vi "canDataSort.vi"() -> ()   [LabVIEW 2023] (continued)
\tFF\tFD\r\n      4002  0CF101A7   00000004    8        68\t00\t97\tCC\t00\t19\t39\tE2\r\n      4002  1FFFFFFF   00000004    8        00\t00\tFF\tFF\tFF\tFF\tFF\tFF\r\n      3993  18F106A7   00000004    8        00\tF7\tFF\tFF\tFF\tFF\tFF\tC0\r\n      3992  1FFFFFFF   00000004    8        00\t00\tFF\tFF\tFF\tFF\tFF\tFF\r\n      3983  0CF102A7   00000004    8        30\t75\tE0\t2E\t80\tFF\tFF\tFD\r\n      3983  0CF101A7   00000004    8        68\t00\t97\tCC\t00\t19\t39\tE1\r\n      3982  1FFFFFFF   00000004    8        00\t00\tFF\tFF\tFF\tFF\tFF\tFF\r\n      3972  1FFFFFFF   00000004    8        00\t00\tFF\tFF\tFF\tFF\tFF\tFF\r\n      3963  0CF102A7   00000004    8        30\t75\tE0\t2E\t80\tFF\tFF\tFD\r\n      4022  1FFFFFFF   00000004    8        00\t00\tFF\tFF\tFF\tFF\tFF\tFF\r\n      4012  1FFFFFFF   00000004    8        00\t20\tFF\tFF\tFF\tFF\tFF\tFF\r\n      4003  0CF102A7   00000004    8        30\t75\tE0\t2E\t80\tFF\tFF\tFD\r\n      4002  0CF101A7   00000004    8        68\t00\t97\tCC\t00\t19\t39\tE2\r\n      4002  1FFFFFFF   00000004    8        00\t00\tFF\tFF\tFF\tFF\tFF\tFF\r\n      3993  18F106A7   00000004    8        00\tF7\tFF\tFF\tFF\tFF\tFF\tC0\r\n      3992  1FFFFFFF   00000004    8        00\t00\tFF\tFF\tFF\tFF\tFF\tFF\r\n      3983  0CF102A7   00000004    8        30\t75\tE0\t2E\t80\tFF\tFF\tFD\r\n      3983  0CF101A7   00000004    8        68\t00\t97\tCC\t00\t19\t39\tE1\r\n      3982  1FFFFFFF   00000004    8        00\t00\tFF\tFF\tFF\tFF\tFF\tFF\r\n      3972  1FFFFFFF   00000004    8        00\t00\tFF\tFF\tFF\tFF\tFF\tFF\r\n      4023  0CF101A7   00000004    8        68\t00\t97\tCC\t00\t19\t39\tE3\r\n      4022  1FFFFFFF   00000004    8        00\t00\tFF\tFF\tFF\tFF\tFF\tFF\r\n      4012  1FFFFFFF   00000004    8        00\t20\tFF\tFF\tFF\tFF\tFF\tFF\r\n      4003  0CF102A7   00000004    8        30\t75\tE0\t2E\t80\tFF\tFF\tFD\r\n      4002  0CF101A7   00000004    8        68\t00\t97\tCC\t00\t19\t39\tE2\r\n      4002  1FFFFFFF   00000004    8        00\t00\tFF\tFF\tFF\tFF\tFF\tFF\r\n      3993  18F106A7   00000004    8        00\tF7\tFF\tFF\tFF\tFF\tFF\tC0\r\n      3992  1FFFFFFF   00000004    8        00\t00\tFF\tFF\tFF\tFF\tFF\tFF\r\n      3983  0CF102A7   00000004    8        30\t75\tE0\t2E\t80\tFF\tFF\tFD\r\n      3983  0CF101A7   00000004    8        68\t00\t97\tCC\t00\t19\t39\tE1\r\n      3982  1FFFFFFF   00000004    8        00\t00\tFF\tFF\tFF\tFF\tFF\tFF\r\n      4023  0CF102A7   00000004    8        30\t75\tE0\t2E\t80\tFF\tFF\tFD\r\n      4023  0CF101A7   00000004    8        68\t00\t97\tCC\t00\t19\t39\tE3\r\n      4022  1FFFFFFF   00000004    8        00\t00\tFF\tFF\tFF\tFF\tFF\tFF\r\n      4012  1FFFFFFF   00000004    8        00\t20\tFF\tFF\tFF\tFF\tFF\tFF\r\n      4003  0CF102A7   00000004    8        30\t75\tE0\t2E\t80\tFF\tFF\tFD\r\n      4002  0CF101A7   00000004    8        68\t00\t97\tCC\t00\t19\t39\tE2\r\n      4002  1FFFFFFF   00000004    8        00\t00\tFF\tFF\tFF\tFF\tFF\tFF\r\n      3993  18F106A7   00000004    8        00\tF7\tFF\tFF\tFF\tFF\tFF\tC0\r\n      3992  1FFFFFFF   00000004    8        00\t00\tFF\tFF\tFF\tFF\tFF\tFF\r\n      3983  0CF102A7   00000004    8        30\t75\tE0\t2E\t80\tFF\tFF\tFD\r\n      3983  0CF101A7   00000004    8        68\t00\t97\tCC\t00\t19\t39\tE1\r\n      4032  1FFFFFFF   00000004    8        00\t00\tFF\tFF\tFF\tFF\tFF\tFF\r\n      4023  0CF102A7   00000004    8        30\t75\tE0\t2E\t80\tFF\tFF\tFD\r\n      4023  0CF101A7   00000004    8        68\t00\t97\tCC\t00\t19\t39\tE3\r\n      4022  1FFFFFFF   00000004    8        00\t00\tFF\tFF\tFF\tFF\tFF\tFF\r\n      4012  1FFFFFFF   00000004    8        00\t20\tFF\tFF\tFF\tFF\tFF\tFF\r\n      4003  0CF102A7   00000004    8        30\t75\tE0\t2E\t80\tFF\tFF\tFD\r\n      4002  0CF101A7   00000004    8        68\t00\t97\tCC\t00\t19\t39\tE2\r\n      4002  1FFFFFFF   00000004    8        00\t00\tFF\tFF\tFF\tFF\tFF\tFF\r\n      3993  18F106A7   00000004    8        00\tF7\tFF\tFF\tFF\tFF\tFF\tC0\r\n      3992  1FFFFFFF   00000004    8        00\t00\tFF\tFF\tFF\tFF\tFF\tFF\r\n      3983  0CF102A7   00000004    8        30\t75\tE0\t2E\t80\tFF\tFF\tFD\r\n      4041  18F11FF0   00000004    8        FF\t3F\t90\t68\t88\t1B\t10\t0C\r\n      4032  1FFFFFFF   00000004    8        00\t00\tFF\tFF\tFF\tFF\tFF\tFF\r\n      4023  0CF102A7   00000004    8        30\t75\tE0\t2E\t80\tFF\tFF\tFD\r\n      4023  0CF101A7   00000004    8        68\t00\t97\tCC\t00\t19\t39\tE3\r\n      4022  1FFFFFFF   00000004    8        00\t00\tFF\tFF\tFF\tFF\tFF\tFF\r\n      4012  1FFFFFFF   00000004    8        00\t20\tFF\tFF\tFF\tFF\tFF\tFF\r\n      4003  0CF102A7   00000004    8        30\t75\tE0\t2E\t80\tFF\tFF\tFD\r\n      4002  0CF101A7   00000004    8        68\t00\t97\tCC\t00\t19\t39\tE2\r\n      4002  1FFFFFFF   00000004    8        00\t00\tFF\tFF\tFF\tFF\tFF\tFF\r\n      3993  18F106A7   00000004    8        00\tF7\tFF\tFF\tFF\tFF\tFF\tC0\r\n      3992  1FFFFFFF   00000004    8        00\t00\tFF\tFF\tFF\tFF\tFF\tFF\r\n      4042  18F120F0   00000004    8        2B\t75\t60\tB1\tB0\t01\tFF\tFF\r\n      4041  18F11FF0   00000004    8        FF\t3F\t90\t68\t88\t1B\t10\t0C\r\n      4032  1FFFFFFF   00000004    8        00\t00\tFF\tFF\tFF\tFF\tFF\tFF\r\n      4023  0CF102A7   00000004    8        30\t75\tE0\t2E\t80\tFF\tFF\tFD\r\n      4023  0CF101A7   00000004    8        68\t00\t97\tCC\t00\t19\t39\tE3\r\n      4022  1FFFFFFF   00000004    8        00\t00\tFF\tFF\tFF\tFF\tFF\tFF\r\n      4012  1FFFFFFF   00000004    8        00\t20\tFF\tFF\tFF\tFF\tFF\tFF\r\n      4003  0CF102A7   00000004    8        30\t75\tE0\t2E\t80\tFF\tFF\tFD\r\n      4002  0CF101A7   00000004    8        68\t00\t97\tCC\t00\t19\t39\tE2\r\n      4002  1FFFFFFF   00000004    8        00\t00\tFF\tFF\tFF\tFF\tFF\tFF\r\n      3993  18F106A7   00000004    8        00\tF7\tFF\tFF\tFF\tFF\tFF\tC0\r\n      4043  0CF101A7   00000004    8        68\t00\t97\tCC\t00\t19\t39\tE4\r\n      4042  18F120F0   00000004    8        2B\t75\t60\tB1\tB0\t01\tFF\tFF\r\n      4041  18F11FF0   00000004    8        FF\t3F\t90\t68\t88\t1B\t10\t0C\r\n      4032  1FFFFFFF   00000004    8        00\t00\tFF\tFF\tFF\tFF\tFF\tFF\r\n      4023  0CF102A7   00000004    8        30\t75\tE0\t2E\t80\tFF\tFF\tFD\r\n      4023  0CF101A7   00000004    8        68\t00\t97\tCC\t00\t19\t39\tE3\r\n      4022  1FFFFFFF   00000004    8        00\t00\tFF\tFF\tFF\tFF\tFF\tFF\r\n      4012  1FFFFFFF   00000004    8        00\t20\tFF\tFF\tFF\tFF\tFF\tFF\r\n      4003  0CF102A7   00000004    8        30\t75\tE0\t2E\t80\tFF\tFF\tFD\r\n      4002  0CF101A7   00000004    8        68\t00\t97\tCC\t00\t19\t39\tE2\r\n      4002  1FFFFFFF   00000004    8        00\t00\tFF\tFF\tFF\tFF\tFF\tFF\r\n      4043  0C3C4D4A   00000004    8        BE\tFF\tFF\t7F\t18\tFF\tFF\t60\r\n      4043  0CF101A7   00000004    8        68\t00\t97\tCC\t00\t19\t39\tE4\r\n      4042  18F120F0   00000004    8        2B\t75\t60\tB1\tB0\t01\tFF\tFF\r\n      4041  18F11FF0   00000004    8        FF\t3F\t90\t68\t88\t1B\t10\t0C\r\n      4032  1FFFFFFF   00000004    8        00\t00\tFF\tFF\tFF\tFF\tFF\tFF\r\n      4023  0CF102A7   00000004    8        30\t75\tE0\t2E\t80\tFF\tFF\tFD\r\n      4023  0CF101A7   00000004    8        68\t00\t97\tCC\t00\t19\t39\tE3\r\n      4022  1FFFFFFF   00000004    8        00\t00\tFF\tFF\tFF\tFF\tFF\tFF\r\n      4012  1FFFFFFF   00000004    8        00\t20\tFF\tFF\tFF\tFF\tFF\tFF\r\n      4003  0CF102A7   00000004    8        30\t75\tE0\t2E\t80\tFF\tFF\tFD\r\n      4002  0CF101A7   00000004    8        68\t00\t97\tCC\t00\t19\t39\tE2\r\n      4044  0CF102A7   00000004    8        30\t75\tE0\t2E\t80\tFF\tFF\tFD\r\n      4043  0C3C4D4A   00000004    8        BE\tFF\tFF\t7F\t18\tFF\tFF\t60\r\n      4043  0CF101A7   00000004    8        68\t00\t97\tCC\t00\t19\t39\tE4\r\n      4042  18F120F0   00000004    8        2B\t75\t60\tB1\tB0\t01\tFF\tFF\r\n      4041  18F11FF0   00000004    8        FF\t3F\t90\t68\t88\t1B\t10\t0C\r\n      4032  1FFFFFFF   00000004    8        00\t00\tFF\tFF\tFF\tFF\tFF\tFF\r\n      4023  0CF102A7   00000004    8        30\t75\tE0\t2E\t80\tFF\tFF\tFD\r\n      4023  0CF101A7   00000004    8        68\t00\t97\tCC\t00\t19\t39\tE3\r\n      4022  1FFFFFFF   00000004    8        00\t00\tFF\tFF\tFF\tFF\tFF\tFF\r\n      4012  1FFFFFFF   00000004    8        00\t20\tFF\tFF\tFF\tFF\tFF\tFF\r\n      4003  0CF102A7   00000004    8        30\t75\tE0\t2E\t80\tFF\tFF\tFD\r\n      4044  0CF103A7   00000004    8        17\t1F\t08\t60\tB1\t1F\t08\t60\r\n      4044  0CF102A7   00000004    8        30\t75\tE0\t2E\t80\tFF\tFF\tFD\r\n      4043  0C3C4D4A   00000004    8        BE\tFF\tFF\t7F\t18\tFF\tFF\t60\r\n      4043  0CF101A7   00000004    8        68\t00\t97\tCC\t00\t19\t39\tE4\r\n      4042  18F120F0   00000004    8        2B\t75\t60\tB1\tB0\t01\tFF\tFF\r\n      4041  18F11FF0   00000004    8        FF\t3F\t90\t68\t88\t1B\t10\t0C\r\n      4032  1FFFFFFF   00000004    8        00\t00\tFF\tFF\tFF\tFF\tFF\tFF\r\n      4023  0CF102A7   00000004    8        30\t75\tE0\t2E\t80\tFF\tFF\tFD\r\n      4023  0CF101A7   00000004    8        68\t00\t97\tCC\t00\t19\t39\tE3\r\n      4022  1FFFFFFF   00000004    8        00\t00\tFF\tFF\tFF\tFF\tFF\tFF\r\n      4012  1FFFFFFF   00000004    8        00\t20\tFF\tFF\tFF\tFF\tFF\tFF\r\n      4045  0CF104A7   00000004    8        F0\t60\t22\tFC\tFF\tFF\tFF\t60\r\n      4044  0CF103A7   00000004    8        17\t1F\t08\t60\tB1\t1F\t08\t60\r\n      4044  0CF102A7   00000004    8        30\t75\tE0\t2E\t80\tFF\tFF\tFD\r\n      4043  0C3C4D4A   00000004    8        BE\tFF\tFF\t7F\t18\tFF\tFF\t60\r\n      4043  0CF101A7   00000004    8        68\t00\t97\tCC\t00\t19\t39\tE4\r\n      4042  18F120F0   00000004    8        2B\t75\t60\tB1\tB0\t01\tFF\tFF\r\n      4041  18F11FF0   00000004    8        FF\t3F\t90\t68\t88\t1B\t10\t0C\r\n      4032  1FFFFFFF   00000004    8        00\t00\tFF\tFF\tFF\tFF\tFF\tFF\r\n      4023  0CF102A7   00000004    8        30\t75\tE0\t2E\t80\tFF\tFF\tFD\r\n      4023  0CF101A7   00000004    8        68\t00\t97\tCC\t00\t19\t39\tE3\r\n      4022  1FFFFFFF   00000004    8        00\t00\tFF\tFF\tFF\tFF\tFF\tFF\r\n      4045  18F106A7   00000004    8        00\tF7\tFF\tFF\tFF\tFF\tFF\tC1\r\n      4045  0CF104A7   00000004    8        F0\t60\t22\tFC\tFF\tFF\tFF\t60\r\n      4044  0CF103A7   00000004    8        17\t1F\t08\t60\tB1\t1F\t08\t60\r\n      4044  0CF102A7   00000004    8        30\t75\tE0\t2E\t80\tFF\tFF\tFD\r\n      4043  0C3C4D4A   00000004    8        BE\tFF\tFF\t7F\t18\tFF\tFF\t60\r\n      4043  0CF101A7   00000004    8        68\t00\t97\tCC\t00\t19\t39\tE4\r\n      4042  18F120F0   00000004    8        2B\t75\t60\tB1\tB0\t01\tFF\tFF\r\n      4041  18F11FF0   00000004    8        FF\t3F\t90\t68\t88\t1B\t10\t0C\r\n      4032  1FFFFFFF   00000004    8        00\t00\tFF\tFF\tFF\tFF\tFF\tFF\r\n      4023  0CF102A7   00000004    8        30\t75\tE0\t2E\t80\tFF\tFF\tFD\r\n      4023  0CF101A7   00000004    8        68\t00\t97\tCC\t00\t19\t39\tE3\r\n      4046  18F121F0   00000004    8        09\t34\t00\t00\tFF\tFF\tB0\t01\r\n      4045  18F106A7   00000004    8        00\tF7\tFF\tFF\tFF\tFF\tFF\tC1\r\n      4045  0CF104A7   00000004    8        F0\t60\t22\tFC\tFF\tFF\tFF\t60\r\n      4044  0CF103A7   00000004    8        17\t1F\t08\t60\tB1\t1F\t08\t60\r\n      4044  0CF102A7   00000004    8        30\t75\tE0\t2E\t80\tFF\tFF\tFD\r\n      4043  0C3C4D4A   00000004    8        BE\tFF\tFF\t7F\t18\tFF\tFF\t60\r\n      4043  0CF101A7   00000004    8        68\t00\t97\tCC\t00\t19\t39\tE4\r\n      4042  18F120F0   00000004    8        2B\t75\t60\tB1\tB0\t01\tFF\tFF\r\n      4041  18F11FF0   00000004    8        FF\t3F\t90\t68\t88\t1B\t10\t0C\r\n      4032  1FFFFFFF   00000004    8        00\t00\tFF\tFF\tFF\tFF\tFF\tFF\r\n      4023  0CF102A7   00000004    8        30\t75\tE0\t2E\t80\tFF\tFF\tFD\r\n      4047  1FFFFFFF   00000004    8        00\t00\tFF\tFF\tFF\tFF\tFF\tFF\r\n      4046  18F121F0   00000004    8        09\t34\t00\t00\tFF\tFF\tB0\t01\r\n      4045  18F106A7   00000004    8        00\tF7\tFF\tFF\tFF\tFF\tFF\tC1\r\n      4045  0CF104A7   00000004    8        F0\t60\t22\tFC\tFF\tFF\tFF\t60\r\n      4044  0CF103A7   00000004    8        17\t1F\t08\t60\tB1\t1F\t08\t60\r\n      4044  0CF102A7   00000004    8        30\t75\tE0\t2E\t80\tFF\tFF\tFD\r\n      4043  0C3C4D4A   00000004    8        BE\tFF\tFF\t7F\t18\tFF\tFF\t60\r\n      4043  0CF101A7   00000004    8        68\t00\t97\tCC\t00\t19\t39\tE4\r\n      4042  18F120F0   00000004    8        2B\t75\t60\tB1\tB0\t01\tFF\tFF\r\n      4041  18F11FF0   00000004    8        FF\t3F\t90\t68\t88\t1B\t10\t0C\r\n      4032  1FFFFFFF   00000004    8        00\t00\tFF\tFF\tFF\tFF\tFF\tFF\r\n      4052  1FFFFFFF   00000004    8        00\t20\tFF\tFF\tFF\tFF\tFF\tFF\r\n      4047  1FFFFFFF   00000004    8        00\t00\tFF\tFF\tFF\tFF\tFF\tFF\r\n      4046  18F121F0   00000004    8        09\t34\t00\t00\tFF\tFF\tB0\t01\r\n      4045  18F106A7   00000004    8        00\tF7\tFF\tFF\tFF\tFF\tFF\tC1\r\n      4045  0CF104A7   00000004    8        F0\t60\t22\tFC\tFF\tFF\tFF\t60\r\n      4044  0CF103A7   00000004    8        17\t1F\t08\t60\tB1\t1F\t08\t60\r\n      4044  0CF102A7   00000004    8        30\t75\tE0\t2E\t80\tFF\tFF\tFD\r\n      4043  0C3C4D4A   00000004    8        BE\tFF\tFF\t7F\t18\tFF\tFF\t60\r\n      4043  0CF101A7   00000004    8        68\t00\t97\tCC\t00\t19\t39\tE4\r\n      4042  18F120F0   00000004    8        2B\t75\t60\tB1\tB0\t01\tFF\tFF\r\n      4041  18F11FF0   00000004    8        FF\t3F\t90\t68\t88\t1B\t10\t0C\r\n      4062  1FFFFFFF   00000004    8        00\t00\tFF\tFF\tFF\tFF\tFF\tFF\r\n      4052  1FFFFFFF   00000004    8        00\t20\tFF\tFF\tFF\tFF\tFF\tFF\r\n      4047  1FFFFFFF   00000004    8        00\t00\tFF\tFF\tFF\tFF\tFF\tFF\r\n      4046  18F121F0   00000004    8        09\t34\t00\t00\tFF\tFF\tB0\t01\r\n      4045  18F106A7   00000004    8        00\tF7\tFF\tFF\tFF\tFF\tFF\tC1\r\n      4045  0CF104A7   00000004    8        F0\t60\t22\tFC\tFF\tFF\tFF\t60\r\n      4044  0CF103A7   00000004    8        17\t1F\t08\t60\tB1\t1F\t08\t60\r\n      4044  0CF102A7   00000004    8        30\t75\tE0\t2E\t80\tFF\tFF\tFD\r\n      4043  0C3C4D4A   00000004    8        BE\tFF\tFF\t7F\t18\tFF\tFF\t60\r\n      4043  0CF101A7   00000004    8        68\t00\t97\tCC\t00\t19\t39\tE4\r\n      4042  18F120F0   00000004    8        2B\t75\t60\tB1\tB0\t01\tFF\tFF\r\n      4063  0CF101A7   00000004    8        68\t00\t97\tCC\t00\t19\t39\tE5\r\n      4062  1FFFFFFF   00000004    8        00\t00\tFF\tFF\tFF\tFF\tFF\tFF\r\n      4052  1FFFFFFF   00000004    8        00\t20\tFF\tFF\tFF\tFF\tFF\tFF\r\n      4047  1FFFFFFF   00000004    8        00\t00\tFF\tFF\tFF\tFF\tFF\tFF\r\n      4046  18F121F0   00000004    8        09\t34\t00\t00\tFF\tFF\tB0\t01\r\n      4045  18F106A7   00000004    8        00\tF7\tFF\tFF\tFF\tFF\tFF\tC1\r\n      4045  0CF104A7   00000004    8        F0\t60\t22\tFC\tFF\tFF\tFF\t60\r\n      4044  0CF103A7   00000004    8        17\t1F\t08\t60\tB1\t1F\t08\t60\r\n      4044  0CF102A7   00000004    8        30\t75\tE0\t2E\t80\tFF\tFF\tFD\r\n      4043  0C3C4D4A   00000004    8        BE\tFF\tFF\t7F\t18\tFF\tFF\t60\r\n      4043  0CF101A7   00000004    8        68\t00\t97\tCC\t00\t19\t39\tE4\r\n      4063  0CF102A7   00000004    8        30\t75\tE0\t2E\t80\tFF\tFF\tFD\r\n      4063  0CF101A7   00000004    8        68\t00\t97\tCC\t00\t19\t39\tE5\r\n      4062  1FFFFFFF   00000004    8        00\t00\tFF\tFF\tFF\tFF\tFF\tFF\r\n      4052  1FFFFFFF   00000004    8        00\t20\tFF\tFF\tFF\tFF\tFF\tFF\r\n      4047  1FFFFFFF   00000004    8        00\t00\tFF\tFF\tFF\tFF\tFF\tFF\r\n      4046  18F121F0   00000004    8        09\t34\t00\t00\tFF\tFF\tB0\t01\r\n      4045  18F106A7   00000004    8        00\tF7\tFF\tFF\tFF\tFF\tFF\tC1\r\n      4045  0CF104A7   00000004    8        F0\t60\t22\tFC\tFF\tFF\tFF\t60\r\n      4044  0CF103A7   00000004    8        17\t1F\t08\t60\tB1\t1F\t08\t60\r\n      4044  0CF102A7   00000004    8        30\t75\tE0\t2E\t80\tFF\tFF\tFD\r\n      4043  0C3C4D4A   00000004    8        BE\tFF\tFF\t7F\t18\tFF\tFF\t60\r\n      4072  1FFFFFFF   00000004    8        00\t20\tFF\tFF\tFF\tFF\tFF\tFF\r\n      4063  0CF102A7   00000004    8        30\t75\tE0\t2E\t80\tFF\tFF\tFD\r\n      4063  0CF101A7   00000004    8        68\t00\t97\tCC\t00\t19\t39\tE5\r\n      4062  1FFFFFFF   00000004    8        00\t00\tFF\tFF\tFF\tFF\tFF\tFF\r\n      4052  1FFFFFFF   00000004    8        00\t20\tFF\tFF\tFF\tFF\tFF\tFF\r\n      4047  1FFFFFFF   00000004    8        00\t00\tFF\tFF\tFF\tFF\tFF\tFF\r\n      4046  18F121F0   00000004    8        09\t34\t00\t00\tFF\tFF\tB0\t01\r\n      4045  18F106A7   00000004    8        00\tF7\tFF\tFF\tFF\tFF\tFF\tC1\r\n      4045  0CF104A7   00000004    8        F0\t60\t22\tFC\tFF\tFF\tFF\t60\r\n      4044  0CF103A7   00000004    8        17\t1F\t08\t60\tB1\t1F\t08\t60\r\n      4044  0CF102A7   00000004    8        30\t75\tE0\t2E\t80\tFF\tFF\tFD\r\n      4082  1FFFFFFF   00000004    8        00\t20\tFF\tFF\tFF\tFF\tFF\tFF\r\n      4072  1FFFFFFF   00000004    8        00\t20\tFF\tFF\tFF\tFF\tFF\tFF\r\n      4063  0CF102A7   00000004    8        30\t75\tE0\t2E\t80\tFF\tFF\tFD\r\n      4063  0CF101A7   00000004    8        68\t00\t97\tCC\t00\t19\t39\tE5\r\n      4062  1FFFFFFF   00000004    8        00\t00\tFF\tFF\tFF\tFF\tFF\tFF\r\n      4052  1FFFFFFF   00000004    8        00\t20\tFF\tFF\tFF\tFF\tFF\tFF\r\n      4047  1FFFFFFF   00000004    8        00\t00\tFF\tFF\tFF\tFF\tFF\tFF\r\n      4046  18F121F0   00000004    8        09\t34\t00\t00\tFF\tFF\tB0\t01\r\n      4045  18F106A7   00000004    8        00\tF7\tFF\tFF\tFF\tFF\tFF\tC1\r\n      4045  0CF104A7   00000004    8        F0\t60\t22\tFC\tFF\tFF\tFF\t60\r\n      4044  0CF103A7   00000004    8        17\t1F\t08\t60\tB1\t1F\t08\t60\r\n      4083  0CF101A7   00000004    8        68\t00\t97\tCC\t00\t19\t39\tE6\r\n      4082  1FFFFFFF   00000004    8        00\t20\tFF\tFF\tFF\tFF\tFF\tFF\r\n      4072  1FFFFFFF   00000004    8        00\t20\tFF\tFF\tFF\tFF\tFF\tFF\r\n      4063  0CF102A7   00000004    8        30\t75\tE0\t2E\t80\tFF\tFF\tFD\r\n      4063  0CF101A7   00000004    8        68\t00\t97\tCC\t00\t19\t39\tE5\r\n      4062  1FFFFFFF   00000004    8        00\t00\tFF\tFF\tFF\tFF\tFF\tFF\r\n      4052  1FFFFFFF   00000004    8        00\t20\tFF\tFF\tFF\tFF\tFF\tFF\r\n      4047  1FFFFFFF   00000004    8        00\t00\tFF\tFF\tFF\tFF\tFF\tFF\r\n      4046  18F121F0   00000004    8        09\t34\t00\t00\tFF\tFF\tB0\t01\r\n      4045  18F106A7   00000004    8        00\tF7\tFF\tFF\tFF\tFF\tFF\tC1\r\n      4045  0CF104A7   00000004    8        F0\t60\t22\tFC\tFF\tFF\tFF\t60\r\n      4083  0CF102A7   00000004    8        30\t75\tE0\t2E\t80\tFF\tFF\tFD\r\n      4083  0CF101A7   00000004    8        68\t00\t97\tCC\t00\t19\t39\tE6\r\n      4082  1FFFFFFF   00000004    8        00\t20\tFF\tFF\tFF\tFF\tFF\tFF\r\n      4072  1FFFFFFF   00000004    8        00\t20\tFF\tFF\tFF\tFF\tFF\tFF\r\n      4063  0CF102A7   00000004    8        30\t75\tE0\t2E\t80\tFF\tFF\tFD\r\n      4063  0CF101A7   00000004    8        68\t00\t97\tCC\t00\t19\t39\tE5\r\n      4062  1FFFFFFF   00000004    8        00\t00\tFF\tFF\tFF\tFF\tFF\tFF\r\n      4052  1FFFFFFF   00000004    8        00\t20\tFF\tFF\tFF\tFF\tFF\tFF\r\n      4047  1FFFFFFF   00000004    8        00\t00\tFF\tFF\tFF\tFF\tFF\tFF\r\n      4046  18F121F0   00000004    8        09\t34\t00\t00\tFF\tFF\tB0\t01\r\n      4045  18F106A7   00000004    8        00\tF7\tFF\tFF\tFF\tFF\tFF\tC1\r\n      4092  1FFFFFFF   00000004    8        00\t00\tFF\tFF\tFF\tFF\tFF\tFF\r\n      4083  0CF102A7   00000004    8        30\t75\tE0\t2E\t80\tFF\tFF\tFD\r\n      4083  0CF101A7   00000004    8        68\t00\t97\tCC\t00\t19\t39\tE6\r\n      4082  1FFFFFFF   00000004    8        00\t20\tFF\tFF\tFF\tFF\tFF\tFF\r\n      4072  1FFFFFFF   00000004    8        00\t20\tFF\tFF\tFF\tFF\tFF\tFF\r\n      4063  0CF102A7   00000004    8        30\t75\tE0\t2E\t80\tFF\tFF\tFD\r\n      4063  0CF101A7   00000004    8        68\t00\t97\tCC\t00\t19\t39\tE5\r\n      4062  1FFFFFFF   00000004    8        00\t00\tFF\tFF\tFF\tFF\tFF\tFF\r\n      4052  1FFFFFFF   00000004    8        00\t20\tFF\tFF\tFF\tFF\tFF\tFF\r\n      4047  1FFFFFFF   00000004    8        00\t00\tFF\tFF\tFF\tFF\tFF\tFF\r\n      4046  18F121F0   00000004    8        09\t34\t00\t00\tFF\tFF\tB0\t01\r\n      4093  18F106A7   00000004    8        00\tF7\tFF\tFF\tFF\tFF\tFF\tC2\r\n      4092  1FFFFFFF   00000004    8        00\t00\tFF\tFF\tFF\tFF\tFF\tFF\r\n      4083  0CF102A7   00000004    8        30\t75\tE0\t2E\t80\tFF\tFF\tFD\r\n      4083  0CF101A7   00000004    8        68\t00\t97\tCC\t00\t19\t39\tE6\r\n      4082  1FFFFFFF   00000004    8        00\t20\tFF\tFF\tFF\tFF\tFF\tFF\r\n      4072  1FFFFFFF   00000004    8        00\t20\tFF\tFF\tFF\tFF\tFF\tFF\r\n      4063  0CF102A7   00000004    8        30\t75\tE0\t2E\t80\tFF\tFF\tFD\r\n      4063  0CF101A7   00000004    8        68\t00\t97\tCC\t00\t19\t39\tE5\r\n      4062  1FFFFFFF   00000004    8        00\t00\tFF\tFF\tFF\tFF\tFF\tFF\r\n      4052  1FFFFFFF   00000004    8        00\t20\tFF\tFF\tFF\tFF\tFF\tFF\r\n      4047  1FFFFFFF   00000004    8        00\t00\tFF\tFF\tFF\tFF\tFF\tFF\r\n      4102  1FFFFFFF   00000004    8        00\t20\tFF\tFF\tFF\tFF\tFF\tFF\r\n      4093  18F106A7   00000004    8        00\tF7\tFF\tFF\tFF\tFF\tFF\tC2\r\n      4092  1FFFFFFF   00000004    8        00\t00\tFF\tFF\tFF\tFF\tFF\tFF\r\n      4083  0CF102A7   00000004    8        30\t75\tE0\t2E\t80\tFF\tFF\tFD\r\n      4083  0CF101A7   00000004    8        68\t00\t97\tCC\t00\t19\t39\tE6\r\n      4082  1FFFFFFF   00000004    8        00\t20\tFF\tFF\tFF\tFF\tFF\tFF\r\n      4072  1FFFFFFF   00000004    8        00\t20\tFF\tFF\tFF\tFF\tFF\tFF\r\n      4063  0CF102A7   00000004    8        30\t75\tE0\t2E\t80\tFF\tFF\tFD\r\n      4063  0CF101A7   00000004    8        68\t00\t97\tCC\t00\t19\t39\tE5\r\n      4062  1FFFFFFF   00000004    8        00\t00\tFF\tFF\tFF\tFF\tFF\tFF\r\n      4052  1FFFFFFF   00000004    8        00\t20\tFF\tFF\tFF\tFF\tFF\tFF\r\n      4103  0CF101A7   00000004    8        68\t00\t97\tCC\t00\t19\t39\tE7\r\n      4102  1FFFFFFF   00000004    8        00\t20\tFF\tFF\tFF\tFF\tFF\tFF\r\n      4093  18F106A7   00000004    8        00\tF7\tFF\tFF\tFF\tFF\tFF\tC2\r\n      4092  1FFFFFFF   00000004    8        00\t00\tFF\tFF\tFF\tFF\tFF\tFF\r\n      4083  0CF102A7   00000004    8        30\t75\tE0\t2E\t80\tFF\tFF\tFD\r\n      4083  0CF101A7   00000004    8        68\t00\t97\tCC\t00\t19\t39\tE6\r\n      4082  1FFFFFFF   00000004    8        00\t20\tFF\tFF\tFF\tFF\tFF\tFF\r\n      4072  1FFFFFFF   00000004    8        00\t20\tFF\tFF\tFF\tFF\tFF\tFF\r\n      4063  0CF102A7   00000004    8        30\t75\tE0\t2E\t80\tFF\tFF\tFD\r\n      4063  0CF101A7   00000004    8        68\t00\t97\tCC\t00\t19\t39\tE5\r\n      4062  1FFFFFFF   00000004    8        00\t00\tFF\tFF\tFF\tFF\tFF\tFF\r\n      4103  0CF102A7   00000004    8        30\t75\tE0\t2E\t80\tFF\tFF\tFD\r\n      4103  0CF101A7   00000004    8        68\t00\t97\tCC\t00\t19\t39\tE7\r\n      4102  1FFFFFFF   00000004    8        00\t20\tFF\tFF\tFF\tFF\tFF\tFF\r\n      4093  18F106A7   00000004    8        00\tF7\tFF\tFF\tFF\tFF\tFF\tC2\r\n      4092  1FFFFFFF   00000004    8        00\t00\tFF\tFF\tFF\tFF\tFF\tFF\r\n      4083  0CF102A7   00000004    8        30\t75\tE0\t2E\t80\tFF\tFF\tFD\r\n      4083  0CF101A7   00000004    8        68\t00\t97\tCC\t00\t19\t39\tE6\r\n      4082  1FFFFFFF   00000004    8        00\t20\tFF\tFF\tFF\tFF\tFF\tFF\r\n      4072  1FFFFFFF   00000004    8        00\t20\tFF\tFF\tFF\tFF\tFF\tFF\r\n      4063  0CF102A7   00000004    8        30\t75\tE0\t2E\t80\tFF\tFF\tFD\r\n      4063  0CF101A7   00000004    8        68\t00\t97\tCC\t00\t19\t39\tE5\r\n      4112  1FFFFFFF   00000004    8        00\t00\tFF\tFF\tFF\tFF\tFF\tFF\r\n      4103  0CF102A7   00000004    8        30\t75\tE0\t2E\t80\tFF\tFF\tFD\r\n      4103  0CF101A7   00000004    8        68\t00\t97\tCC\t00\t19\t39\tE7\r\n      4102  1FFFFFFF   00000004    8        00\t20\tFF\tFF\tFF\tFF\tFF\tFF\r\n      4093  18F106A7   00000004    8        00\tF7\tFF\tFF\tFF\tFF\tFF\tC2\r\n      4092  1FFFFFFF   00000004    8        00\t00\tFF\tFF\tFF\tFF\tFF\tFF\r\n      4083  0CF102A7   00000004    8        30\t75\tE0\t2E\t80\tFF\tFF\tFD\r\n      4083  0CF101A7   00000004    8        68\t00\t97\tCC\t00\t19\t39\tE6\r\n      4082  1FFFFFFF   00000004    8        00\t20\tFF\tFF\tFF\tFF\tFF\tFF\r\n      4072  1FFFFFFF   00000004    8        00\t20\tFF\tFF\tFF\tFF\tFF\tFF\r\n      4063  0CF102A7   00000004    8        30\t75\tE0\t2E\t80\tFF\tFF\tFD\r\n      4122  1FFFFFFF   00000004    8        00\t20\tFF\tFF\tFF\tFF\tFF\tFF\r\n      4112  1FFFFFFF   00000004    8        00\t00\tFF\tFF\tFF\tFF\tFF\tFF\r\n      4103  0CF102A7   00000004    8        30\t75\tE0\t2E\t80\tFF\tFF\tFD\r\n      4103  0CF101A7   00000004    8        68\t00\t97\tCC\t00\t19\t39\tE7\r\n      4102  1FFFFFFF   00000004    8        00\t20\tFF\tFF\tFF\tFF\tFF\tFF\r\n      4093  18F106A7   00000004    8        00\tF7\tFF\tFF\tFF\tFF\tFF\tC2\r\n      4092  1FFFFFFF   00000004    8        00\t00\tFF\tFF\tFF\tFF\tFF\tFF\r\n      4083  0CF102A7   00000004    8        30\t75\tE0\t2E\t80\tFF\tFF\tFD\r\n      4083  0CF101A7   00000004    8        68\t00\t97\tCC\t00\t19\t39\tE6\r\n      4082  1FFFFFFF   00000004    8        00\t20\tFF\tFF\tFF\tFF\tFF\tFF\r\n      4072  1FFFFFFF   00000004    8        00\t20\tFF\tFF\tFF\tFF\tFF\tFF\r\n      4123  0CF101A7   00000004    8        68\t00\t97\tCC\t00\t19\t39\tE8\r\n      4122  1FFFFFFF   00000004    8        00\t20\tFF\tFF\tFF\tFF\tFF\tFF\r\n      4112  1FFFFFFF   00000004    8        00\t00\tFF\tFF\tFF\tFF\tFF\tFF\r\n      4103  0CF102A7   00000004    8        30\t75\tE0\t2E\t80\tFF\tFF\tFD\r\n      4103  0CF101A7   00000004    8        68\t00\t97\tCC\t00\t19\t39\tE7\r\n      4102  1FFFFFFF   00000004    8        00\t20\tFF\tFF\tFF\tFF\tFF\tFF\r\n      4093  18F106A7   00000004    8        00\tF7\tFF\tFF\tFF\tFF\tFF\tC2\r\n      4092  1FFFFFFF   00000004    8        00\t00\tFF\tFF\tFF\tFF\tFF\tFF\r\n      4083  0CF102A7   00000004    8        30\t75\tE0\t2E\t80\tFF\tFF\tFD\r\n      4083  0CF101A7   00000004    8        68\t00\t97\tCC\t00\t19\t39\tE6\r\n      4082  1FFFFFFF   00000004    8        00\t20\tFF\tFF\tFF\tFF\tFF\tFF\r\n      4123  0CF102A7   00000004    8        30\t75\tE0\t2E\t80\tFF\tFF\tFD\r\n      4123  0CF101A7   00000004    8        68\t00\t97\tCC\t00\t19\t39\tE8\r\n      4122  1FFFFFFF   00000004    8        00\t20\tFF\tFF\tFF\tFF\tFF\tFF\r\n      4112  1FFFFFFF   00000004    8        00\t00\tFF\tFF\tFF\tFF\tFF\tFF\r\n      4103  0CF102A7   00000004    8        30\t75\tE0\t2E\t80\tFF\tFF\tFD\r\n      4103  0CF101A7   00000004    8        68\t00\t97\tCC\t00\t19\t39\tE7\r\n      4102  1FFFFFFF   00000004    8        00\t20\tFF\tFF\tFF\tFF\tFF\tFF\r\n      4093  18F106A7   00000004    8        00\tF7\tFF\tFF\tFF\tFF\tFF\tC2\r\n      4092  1FFFFFFF   00000004    8        00\t00\tFF\tFF\tFF\tFF\tFF\tFF\r\n      4083  0CF102A7   00000004    8        30\t75\tE0\t2E\t80\tFF\tFF\tFD\r\n      4083  0CF101A7   00000004    8        68\t00\t97\tCC\t00\t19\t39\tE6\r\n      4132  1FFFFFFF   00000004    8        00\t20\tFF\tFF\tFF\tFF\tFF\tFF\r\n      4123  0CF102A7   00000004    8        30\t75\tE0\t2E\t80\tFF\tFF\tFD\r\n      4123  0CF101A7   00000004    8        68\t00\t97\tCC\t00\t19\t39\tE8\r\n      4122  1FFFFFFF   00000004    8        00\t20\tFF\tFF\tFF\tFF\tFF\tFF\r\n      4112  1FFFFFFF   00000004    8        00\t00\tFF\tFF\tFF\tFF\tFF\tFF\r\n      4103  0CF102A7   00000004    8        30\t75\tE0\t2E\t80\tFF\tFF\tFD\r\n      4103  0CF101A7   00000004    8        68\t00\t97\tCC\t00\t19\t39\tE7\r\n      4102  1FFFFFFF   00000004    8        00\t20\tFF\tFF\tFF\tFF\tFF\tFF\r\n      4093  18F106A7   00000004    8        00\tF7\tFF\tFF\tFF\tFF\tFF\tC2\r\n      4092  1FFFFFFF   00000004    8        00\t00\tFF\tFF\tFF\tFF\tFF\tFF\r\n      4083  0CF102A7   00000004    8        30\t75\tE0\t2E\t80\tFF\tFF\tFD\r\n      4141  18F11FF0   00000004    8        FF\t3F\t90\t68\t88\t1B\t10\t1C\r\n      4132  1FFFFFFF   00000004    8        00\t20\tFF\tFF\tFF\tFF\tFF\tFF\r\n      4123  0CF102A7   00000004    8        30\t75\tE0\t2E\t80\tFF\tFF\tFD\r\n      4123  0CF101A7   00000004    8        68\t00\t97\tCC\t00\t19\t39\tE8\r\n      4122  1FFFFFFF   00000004    8        00\t20\tFF\tFF\tFF\tFF\tFF\tFF\r\n      4112  1FFFFFFF   00000004    8        00\t00\tFF\tFF\tFF\tFF\tFF\tFF\r\n      4103  0CF102A7   00000004    8        30\t75\tE0\t2E\t80\tFF\tFF\tFD\r\n      4103  0CF101A7   00000004    8        68\t00\t97\tCC\t00\t19\t39\tE7\r\n      4102  1FFFFFFF   00000004    8        00\t20\tFF\tFF\tFF\tFF\tFF\tFF\r\n      4093  18F106A7   00000004    8        00\tF7\tFF\tFF\tFF\tFF\tFF\tC2\r\n      4092  1FFFFFFF   00000004    8        00\t00\tFF\tFF\tFF\tFF\tFF\tFF\r\n      4142  18F120F0   00000004    8        2B\t75\t60\tB1\tB0\t01\tFF\tFF\r\n      4141  18F11FF0   00000004    8        FF\t3F\t90\t68\t88\t1B\t10\t1C\r\n      4132  1FFFFFFF   00000004    8        00\t20\tFF\tFF\tFF\tFF\tFF\tFF\r\n      4123  0CF102A7   00000004    8        30\t75\tE0\t2E\t80\tFF\tFF\tFD\r\n      4123  0CF101A7   00000004    8        68\t00\t97\tCC\t00\t19\t39\tE8\r\n      4122  1FFFFFFF   00000004    8        00\t20\tFF\tFF\tFF\tFF\tFF\tFF\r\n      4112  1FFFFFFF   00000004    8        00\t00\tFF\tFF\tFF\tFF\tFF\tFF\r\n      4103  0CF102A7   00000004    8        30\t75\tE0\t2E\t80\tFF\tFF\tFD\r\n      4103  0CF101A7   00000004    8        68\t00\t97\tCC\t00\t19\t39\tE7\r\n      4102  1FFFFFFF   00000004    8        00\t20\tFF\tFF\tFF\tFF\tFF\tFF\r\n      4093  18F106A7   00000004    8        00\tF7\tFF\tFF\tFF\tFF\tFF\tC2\r\n      4143  0CF101A7   00000004    8        68\t00\t97\tCC\t00\t19\t39\tE9\r\n      4142  18F120F0   00000004    8        2B\t75\t60\tB1\tB0\t01\tFF\tFF\r\n      4141  18F11FF0   00000004    8        FF\t3F\t90\t68\t88\t1B\t10\t1C\r\n      4132  1FFFFFFF   00000004    8        00\t20\tFF\tFF\tFF\tFF\tFF\tFF\r\n      4123  0CF102A7   00000004    8        30\t75\tE0\t2E\t80\tFF\tFF\tFD\r\n      4123  0CF101A7   00000004    8        68\t00\t97\tCC\t00\t19\t39\tE8\r\n      4122  1FFFFFFF   00000004    8        00\t20\tFF\tFF\tFF\tFF\tFF\tFF\r\n      4112  1FFFFFFF   00000004    8        00\t00\tFF\tFF\tFF\tFF\tFF\tFF\r\n      4103  0CF102A7   00000004    8        30\t75\tE0\t2E\t80\tFF\tFF\tFD\r\n      4103  0CF101A7   00000004    8        68\t00\t97\tCC\t00\t19\t39\tE7\r\n      4102  1FFFFFFF   00000004    8        00\t20\tFF\tFF\tFF\tFF\tFF\tFF\r\n      4143  0C3C4D4A   00000004    8        BE\tFF\tFF\t7F\t18\tFF\tFF\t61\r\n      4143  0CF101A7   00000004    8        68\t00\t97\tCC\t00\t19\t39\tE9\r\n      4142  18F120F0   00000004    8        2B\t75\t60\tB1\tB0\t01\tFF\tFF\r\n      4141  18F11FF0   00000004    8        FF\t3F\t90\t68\t88\t1B\t10\t1C\r\n      4132  1FFFFFFF   00000004    8        00\t20\tFF\tFF\tFF\tFF\tFF\tFF\r\n      4123  0CF102A7   00000004    8        30\t75\tE0\t2E\t80\tFF\tFF\tFD\r\n      4123  0CF101A7   00000004    8        68\t00\t97\tCC\t00\t19\t39\tE8\r\n      4122  1FFFFFFF   00000004    8        00\t20\tFF\tFF\tFF\tFF\tFF\tFF\r\n      4112  1FFFFFFF   00000004    8        00\t00\tFF\tFF\tFF\tFF\tFF\tFF\r\n      4103  0CF102A7   00000004    8        30\t75\tE0\t2E\t80\tFF\tFF\tFD\r\n      4103  0CF101A7   00000004    8        68\t00\t97\tCC\t00\t19\t39\tE7\r\n      4144  0CF102A7   00000004    8        30\t75\tE0\t2E\t80\tFF\tFF\tFD\r\n      4143  0C3C4D4A   00000004    8        BE\tFF\tFF\t7F\t18\tFF\tFF\t61\r\n      4143  0CF101A7   00000004    8        68\t00\t97\tCC\t00\t19\t39\tE9\r\n      4142  18F120F0   00000004    8        2B\t75\t60\tB1\tB0\t01\tFF\tFF\r\n      4141  18F11FF0   00000004    8        FF\t3F\t90\t68\t88\t1B\t10\t1C\r\n      4132  1FFFFFFF   00000004    8        00\t20\tFF\tFF\tFF\tFF\tFF\tFF\r\n      4123  0CF102A7   00000004    8        30\t75\tE0\t2E\t80\tFF\tFF\tFD\r\n      4123  0CF101A7   00000004    8        68\t00\t97\tCC\t00\t19\t39\tE8\r\n      4122  1FFFFFFF   00000004    8        00\t20\tFF\tFF\tFF\tFF\tFF\tFF\r\n      4112  1FFFFFFF   00000004    8        00\t00\tFF\tFF\tFF\tFF\tFF\tFF\r\n      4103  0CF102A7   00000004    8        30\t75\tE0\t2E\t80\tFF\tFF\tFD\r\n      4144  0CF103A7   00000004    8        17\t1F\t08\t60\tB1\t1F\t08\t61\r\n      4144  0CF102A7   00000004    8        30\t75\tE0\t2E\t80\tFF\tFF\tFD\r\n      4143  0C3C4D4A   00000004    8        BE\tFF\tFF\t7F\t18\tFF\tFF\t61\r\n      4143  0CF101A7   00000004    8        68\t00\t97\tCC\t00\t19\t39\tE9\r\n      4142  18F120F0   00000004    8        2B\t75\t60\tB1\tB0\t01\tFF\tFF\r\n      4141  18F11FF0   00000004    8        FF\t3F\t90\t68\t88\t1B\t10\t1C\r\n      4132  1FFFFFFF   00000004    8        00\t20\tFF\tFF\tFF\tFF\tFF\tFF\r\n      4123  0CF102A7   00000004    8        30\t75\tE0\t2E\t80\tFF\tFF\tFD\r\n      4123  0CF101A7   00000004    8        68\t00\t97\tCC\t00\t19\t39\tE8\r\n      4122  1FFFFFFF   00000004    8        00\t20\tFF\tFF\tFF\tFF\tFF\tFF\r\n      4112  1FFFFFFF   00000004    8        00\t00\tFF\tFF\tFF\tFF\tFF\tFF\r\n      4145  0CF104A7   00000004    8        F0\t60\t22\tFC\tFF\tFF\tFF\t61\r\n      4144  0CF103A7   00000004    8        17\t1F\t08\t60\tB1\t1F\t08\t61\r\n      4144  0CF102A7   00000004    8        30\t75\tE0\t2E\t80\tFF\tFF\tFD\r\n      4143  0C3C4D4A   00000004    8        BE\tFF\tFF\t7F\t18\tFF\tFF\t61\r\n      4143  0CF101A7   00000004    8        68\t00\t97\tCC\t00\t19\t39\tE9\r\n      4142  18F120F0   00000004    8        2B\t75\t60\tB1\tB0\t01\tFF\tFF\r\n      4141  18F11FF0   00000004    8        FF\t3F\t90\t68\t88\t1B\t10\t1C\r\n      4132  1FFFFFFF   00000004    8        00\t20\tFF\tFF\tFF\tFF\tFF\tFF\r\n      4123  0CF102A7   00000004    8        30\t75\tE0\t2E\t80\tFF\tFF\tFD\r\n      4123  0CF101A7   00000004    8        68\t00\t97\tCC\t00\t19\t39\tE8\r\n      4122  1FFFFFFF   00000004    8        00\t20\tFF\tFF\tFF\tFF\tFF\tFF\r\n      4145  18F106A7   00000004    8        00\tF7\tFF\tFF\tFF\tFF\tFF\tC3\r\n      4145  0CF104A7   00000004    8        F0\t60\t22\tFC\tFF\tFF\tFF\t61\r\n      4144  0CF103A7   00000004    8        17\t1F\t08\t60\tB1\t1F\t08\t61\r\n      4144  0CF102A7   00000004    8        30\t75\tE0\t2E\t80\tFF\tFF\tFD\r\n      4143  0C3C4D4A   00000004    8        BE\tFF\tFF\t7F\t18\tFF\tFF\t61\r\n      4143  0CF101A7   00000004    8        68\t00\t97\tCC\t00\t19\t39\tE9\r\n      4142  18F120F0   00000004    8        2B\t75\t60\tB1\tB0\t01\tFF\tFF\r\n      4141  18F11FF0   00000004    8        FF\t3F\t90\t68\t88\t1B\t10\t1C\r\n      4132  1FFFFFFF   00000004    8        00\t20\tFF\tFF\tFF\tFF\tFF\tFF\r\n      4123  0CF102A7   00000004    8        30\t75\tE0\t2E\t80\tFF\tFF\tFD\r\n      4123  0CF101A7   00000004    8        68\t00\t97\tCC\t00\t19\t39\tE8\r\n      4146  18F108A7   00000004    8        F0\t00\t00\tFF\tFF\tFF\tFF\t46\r\n      4145  18F106A7   00000004    8        00\tF7\tFF\tFF\tFF\tFF\tFF\tC3\r\n      4145  0CF104A7   00000004    8        F0\t60\t22\tFC\tFF\tFF\tFF\t61\r\n      4144  0CF103A7   00000004    8        17\t1F\t08\t60\tB1\t1F\t08\t61\r\n      4144  0CF102A7   00000004    8        30\t75\tE0\t2E\t80\tFF\tFF\tFD\r\n      4143  0C3C4D4A   00000004    8        BE\tFF\tFF\t7F\t18\tFF\tFF\t61\r\n      4143  0CF101A7   00000004    8        68\t00\t97\tCC\t00\t19\t39\tE9\r\n      4142  18F120F0   00000004    8        2B\t75\t60\tB1\tB0\t01\tFF\tFF\r\n      4141  18F11FF0   00000004    8        FF\t3F\t90\t68\t88\t1B\t10\t1C\r\n      4132  1FFFFFFF   00000004    8        00\t20\tFF\tFF\tFF\tFF\tFF\tFF\r\n      4123  0CF102A7   00000004    8        30\t75\tE0\t2E\t80\tFF\tFF\tFD\r\n      4146  18F121F0   00000004    8        09\t34\t00\t00\tFF\tFF\tB0\t01\r\n      4146  18F108A7   00000004    8        F0\t00\t00\tFF\tFF\tFF\tFF\t46\r\n      4145  18F106A7   00000004    8        00\tF7\tFF\tFF\tFF\tFF\tFF\tC3\r\n      4145  0CF104A7   00000004    8        F0\t60\t22\tFC\tFF\tFF\tFF\t61\r\n      4144  0CF103A7   00000004    8        17\t1F\t08\t60\tB1\t1F\t08\t61\r\n      4144  0CF102A7   00000004    8        30\t75\tE0\t2E\t80\tFF\tFF\tFD\r\n      4143  0C3C4D4A   00000004    8        BE\tFF\tFF\t7F\t18\tFF\tFF\t61\r\n      4143  0CF101A7   00000004    8        68\t00\t97\tCC\t00\t19\t39\tE9\r\n      4142  18F120F0   00000004    8        2B\t75\t60\tB1\tB0\t01\tFF\tFF\r\n      4141  18F11FF0   00000004    8        FF\t3F\t90\t68\t88\t1B\t10\t1C\r\n      4132  1FFFFFFF   00000004    8        00\t20\tFF\tFF\tFF\tFF\tFF\tFF\r\n      4147  18FEF117   00000004    8        F7\t97\tCC\tCF\tFF\tFF\tFF\tFF\r\n      4146  18F121F0   00000004    8        09\t34\t00\t00\tFF\tFF\tB0\t01\r\n      4146  18F108A7   00000004    8        F0\t00\t00\tFF\tFF\tFF\tFF\t46\r\n      4145  18F106A7   00000004    8        00\tF7\tFF\tFF\tFF\tFF\tFF\tC3\r\n      4145  0CF104A7   00000004    8        F0\t60\t22\tFC\tFF\tFF\tFF\t61\r\n      4144  0CF103A7   00000004    8        17\t1F\t08\t60\tB1\t1F\t08\t61\r\n      4144  0CF102A7   00000004    8        30\t75\tE0\t2E\t80\tFF\tFF\tFD\r\n      4143  0C3C4D4A   00000004    8        BE\tFF\tFF\t7F\t18\tFF\tFF\t61\r\n      4143  0CF101A7   00000004    8        68\t00\t97\tCC\t00\t19\t39\tE9\r\n      4142  18F120F0   00000004    8        2B\t75\t60\tB1\tB0\t01\tFF\tFF\r\n      4141  18F11FF0   00000004    8        FF\t3F\t90\t68\t88\t1B\t10\t1C\r\n      4148  1FFFFFFF   00000004    8        00\t20\tFF\tFF\tFF\tFF\tFF\tFF\r\n      4147  18FEF117   00000004    8        F7\t97\tCC\tCF\tFF\tFF\tFF\tFF\r\n      4146  18F121F0   00000004    8        09\t34\t00\t00\tFF\tFF\tB0\t01\r\n      4146  18F108A7   00000004    8        F0\t00\t00\tFF\tFF\tFF\tFF\t46\r\n      4145  18F106A7   00000004    8        00\tF7\tFF\tFF\tFF\tFF\tFF\tC3\r\n      4145  0CF104A7   00000004    8        F0\t60\t22\tFC\tFF\tFF\tFF\t61\r\n      4144  0CF103A7   00000004    8        17\t1F\t08\t60\tB1\t1F\t08\t61\r\n      4144  0CF102A7   00000004    8        30\t75\tE0\t2E\t80\tFF\tFF\tFD\r\n      4143  0C3C4D4A   00000004    8        BE\tFF\tFF\t7F\t18\tFF\tFF\t61\r\n      4143  0CF101A7   00000004    8        68\t00\t97\tCC\t00\t19\t39\tE9\r\n      4142  18F120F0   00000004    8        2B\t75\t60\tB1\tB0\t01\tFF\tFF\r\n      4152  1FFFFFFF   00000004    8        00\t20\tFF\tFF\tFF\tFF\tFF\tFF\r\n      4148  1FFFFFFF   00000004    8        00\t20\tFF\tFF\tFF\tFF\tFF\tFF\r\n      4147  18FEF117   00000004    8        F7\t97\tCC\tCF\tFF\tFF\tFF\tFF\r\n      4146  18F121F0   00000004    8        09\t34\t00\t00\tFF\tFF\tB0\t01\r\n      4146  18F108A7   00000004    8        F0\t00\t00\tFF\tFF\tFF\tFF\t46\r\n      4145  18F106A7   00000004    8        00\tF7\tFF\tFF\tFF\tFF\tFF\tC3\r\n      4145  0CF104A7   00000004    8        F0\t60\t22\tFC\tFF\tFF\tFF\t61\r\n      4144  0CF103A7   00000004    8        17\t1F\t08\t60\tB1\t1F\t08\t61\r\n      4144  0CF102A7   00000004    8        30\t75\tE0\t2E\t80\tFF\tFF\tFD\r\n      4143  0C3C4D4A   00000004    8        BE\tFF\tFF\t7F\t18\tFF\tFF\t61\r\n      4143  0CF101A7   00000004    8        68\t00\t97\tCC\t00\t19\t39\tE9\r\n      4162  1FFFFFFF   00000004    8        00\t20\tFF\tFF\tFF\tFF\tFF\tFF\r\n      4152  1FFFFFFF   00000004    8        00\t20\tFF\tFF\tFF\tFF\tFF\tFF\r\n      4148  1FFFFFFF   00000004    8        00\t20\tFF\tFF\tFF\tFF\tFF\tFF\r\n      4147  18FEF117   00000004    8        F7\t97\tCC\tCF\tFF\tFF\tFF\tFF\r\n      4146  18F121F0   00000004    8        09\t34\t00\t00\tFF\tFF\tB0\t01\r\n      4146  18F108A7   00000004    8        F0\t00\t00\tFF\tFF\tFF\tFF\t46\r\n      4145  18F106A7   00000004    8        00\tF7\tFF\tFF\tFF\tFF\tFF\tC3\r\n      4145  0CF104A7   00000004    8        F0\t60\t22\tFC\tFF\tFF\tFF\t61\r\n      4144  0CF103A7   00000004    8        17\t1F\t
